vi "PROXY_alternate_colors_by_timestamp_difference.vi"(6 "message_history_buffer":T1[](array[typedef]), 8 "error_in":errorcluster, 11 "listbox_ref":refnum<vi>) -> (0 "error_out":errorcluster)   [LabVIEW 2020]
uses:
  FGV/DIAGNOSTICS_message_history_buffer/PROXY_DIAGNOSTICS_message_history_buffer_all_info.ctl
  STATION/station.ctl
  _misc/DIAGNOSTICS_message_type.ctl
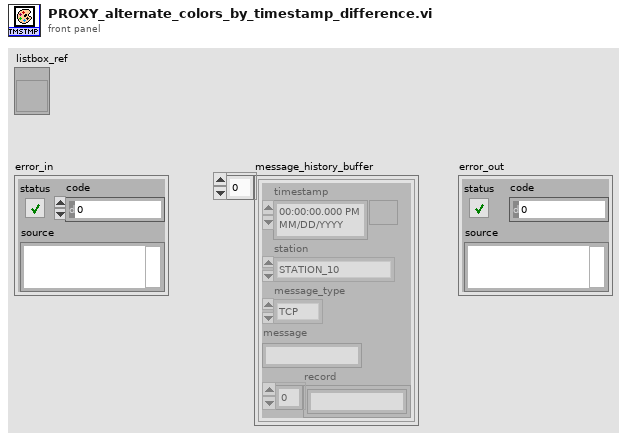
[diagram p1: front panel]
types:
  T1 = typedef "PROXY_DIAGNOSTICS_message_history_buffer_all_info.ctl" = cluster{"timestamp":timestamp, "station":T2, "message_type":T3, "message":string, "record":string[]}
  T2 = typedef "station.ctl" = enum16{"STATION_10", "STATION_20", "STATION_30", "STATION_40", "STATION_50", "STATION_60", "STATION_70", "STATION_80", "STATION_90", "STATION_100", "STATION_110", "STATION_120", "STATION_165", "MAIN"}
  T3 = typedef "DIAGNOSTICS_message_type.ctl" = enum16{"TCP", "SQL"}
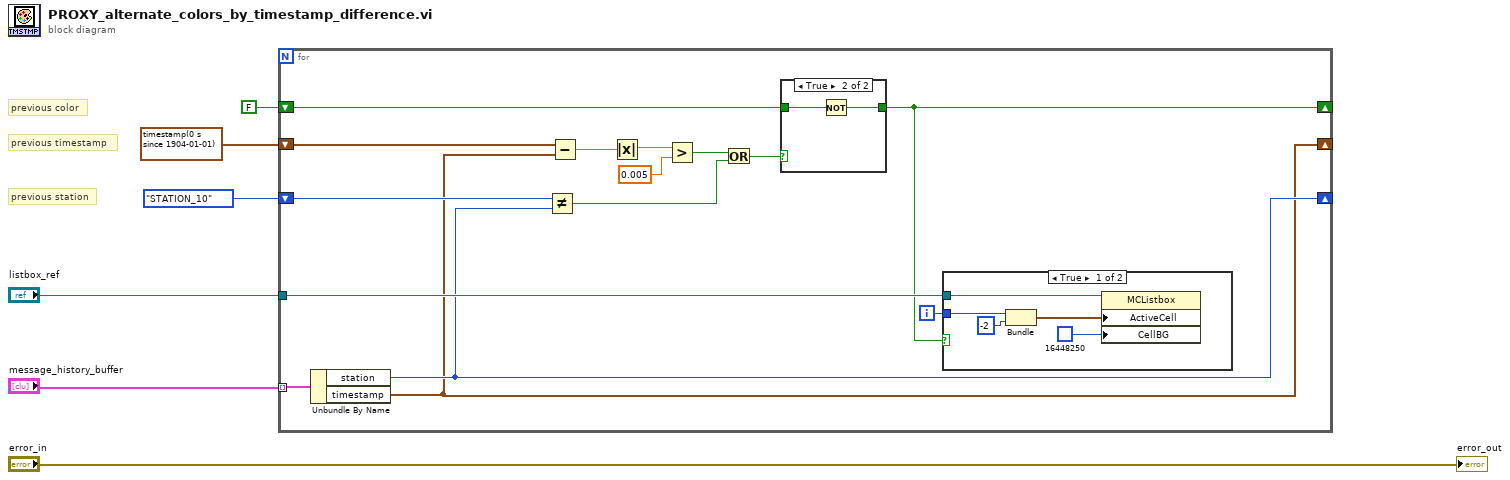
[diagram p0: block diagram]
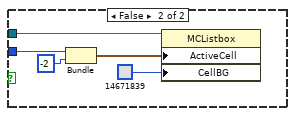
[diagram p3: hidden frame]
diagram:
  # "previous station"
  # "previous timestamp"
  # "previous color"
  n1 = for {
    tunnel: "listbox_ref" -> [w21]
    tunnel: "message_history_buffer" -> [w19] mode=indexing
    shift-right: [w7] -> _
    shift-left: FALSE -> [w10]
    shift-right: [w8] -> _
    shift-left: timestamp(0 s since 1904-01-01) ("timestamp") -> [w9]
    shift-right: [w17] -> _
    shift-left: station."STATION_10" ("station") -> [w18]
    i -> [w20]
    n2 = Unbundle By Name(w19) -> ("station"=w17:T2, "timestamp"=w8:timestamp)
    n3 = Not Equal?(x=w18, y=w17) -> (x != y?=w12:bool)
    n4 = Subtract(x=w9, y=w8) -> (x-y=w16:dbl)
    n5 = Absolute Value(x=w16) -> (abs(x)=w15:dbl)
    n6 = Greater?(x=w15, y=0.005) -> (0:w13:bool)
    n7 = Or(x=w13, y=w12) -> (x .or. y?=w11:bool)
    n8 = case shown="True" w11 {
      tunnel: w10 -> [w22 w24]
      tunnel: [w22 w23] -> w7
      frame False {
      }
      frame True {
        n9 = Not(x=w24) -> (.not. x?=w23:bool)
      }
    }
    n10 = case shown="True" w7 {
      tunnel: w21 -> [w25 w34]
      tunnel: w20 -> [w26 w30]
      frame True {
        n11 = Bundle(w26, -2) -> (w28:cluster{i32, i32})  [unwired: 1 in]
        n12 = property on="Property Node" class="MCListbox"(reference=w25, "ActiveCell"=w28, "CellBG"=u32 16448250) -> ()  [unwired: 1 in, 2 out]
      }
      frame False {
        n13 = Bundle(w30, -2) -> (w32:cluster{i32, i32})  [unwired: 1 in]
        n14 = property on="Property Node" class="MCListbox"(reference=w34, "ActiveCell"=w32, "CellBG"=u32 14671839) -> ()  [unwired: 1 in, 2 out]
      }
    }
  }
  "error_out" <- "error_in"
